vi "Simulator Thresholding.vi"(4 "RAW SICK":i16[](array[numeric]), 6 "SICK Threshold":i16, 7 "Current compass in sectors":i16) -> (0 "Actual SICK (old format)":i16[](array[numeric]), 2 "Binary SICK":i16[](array[numeric]))   [LabVIEW 2009]
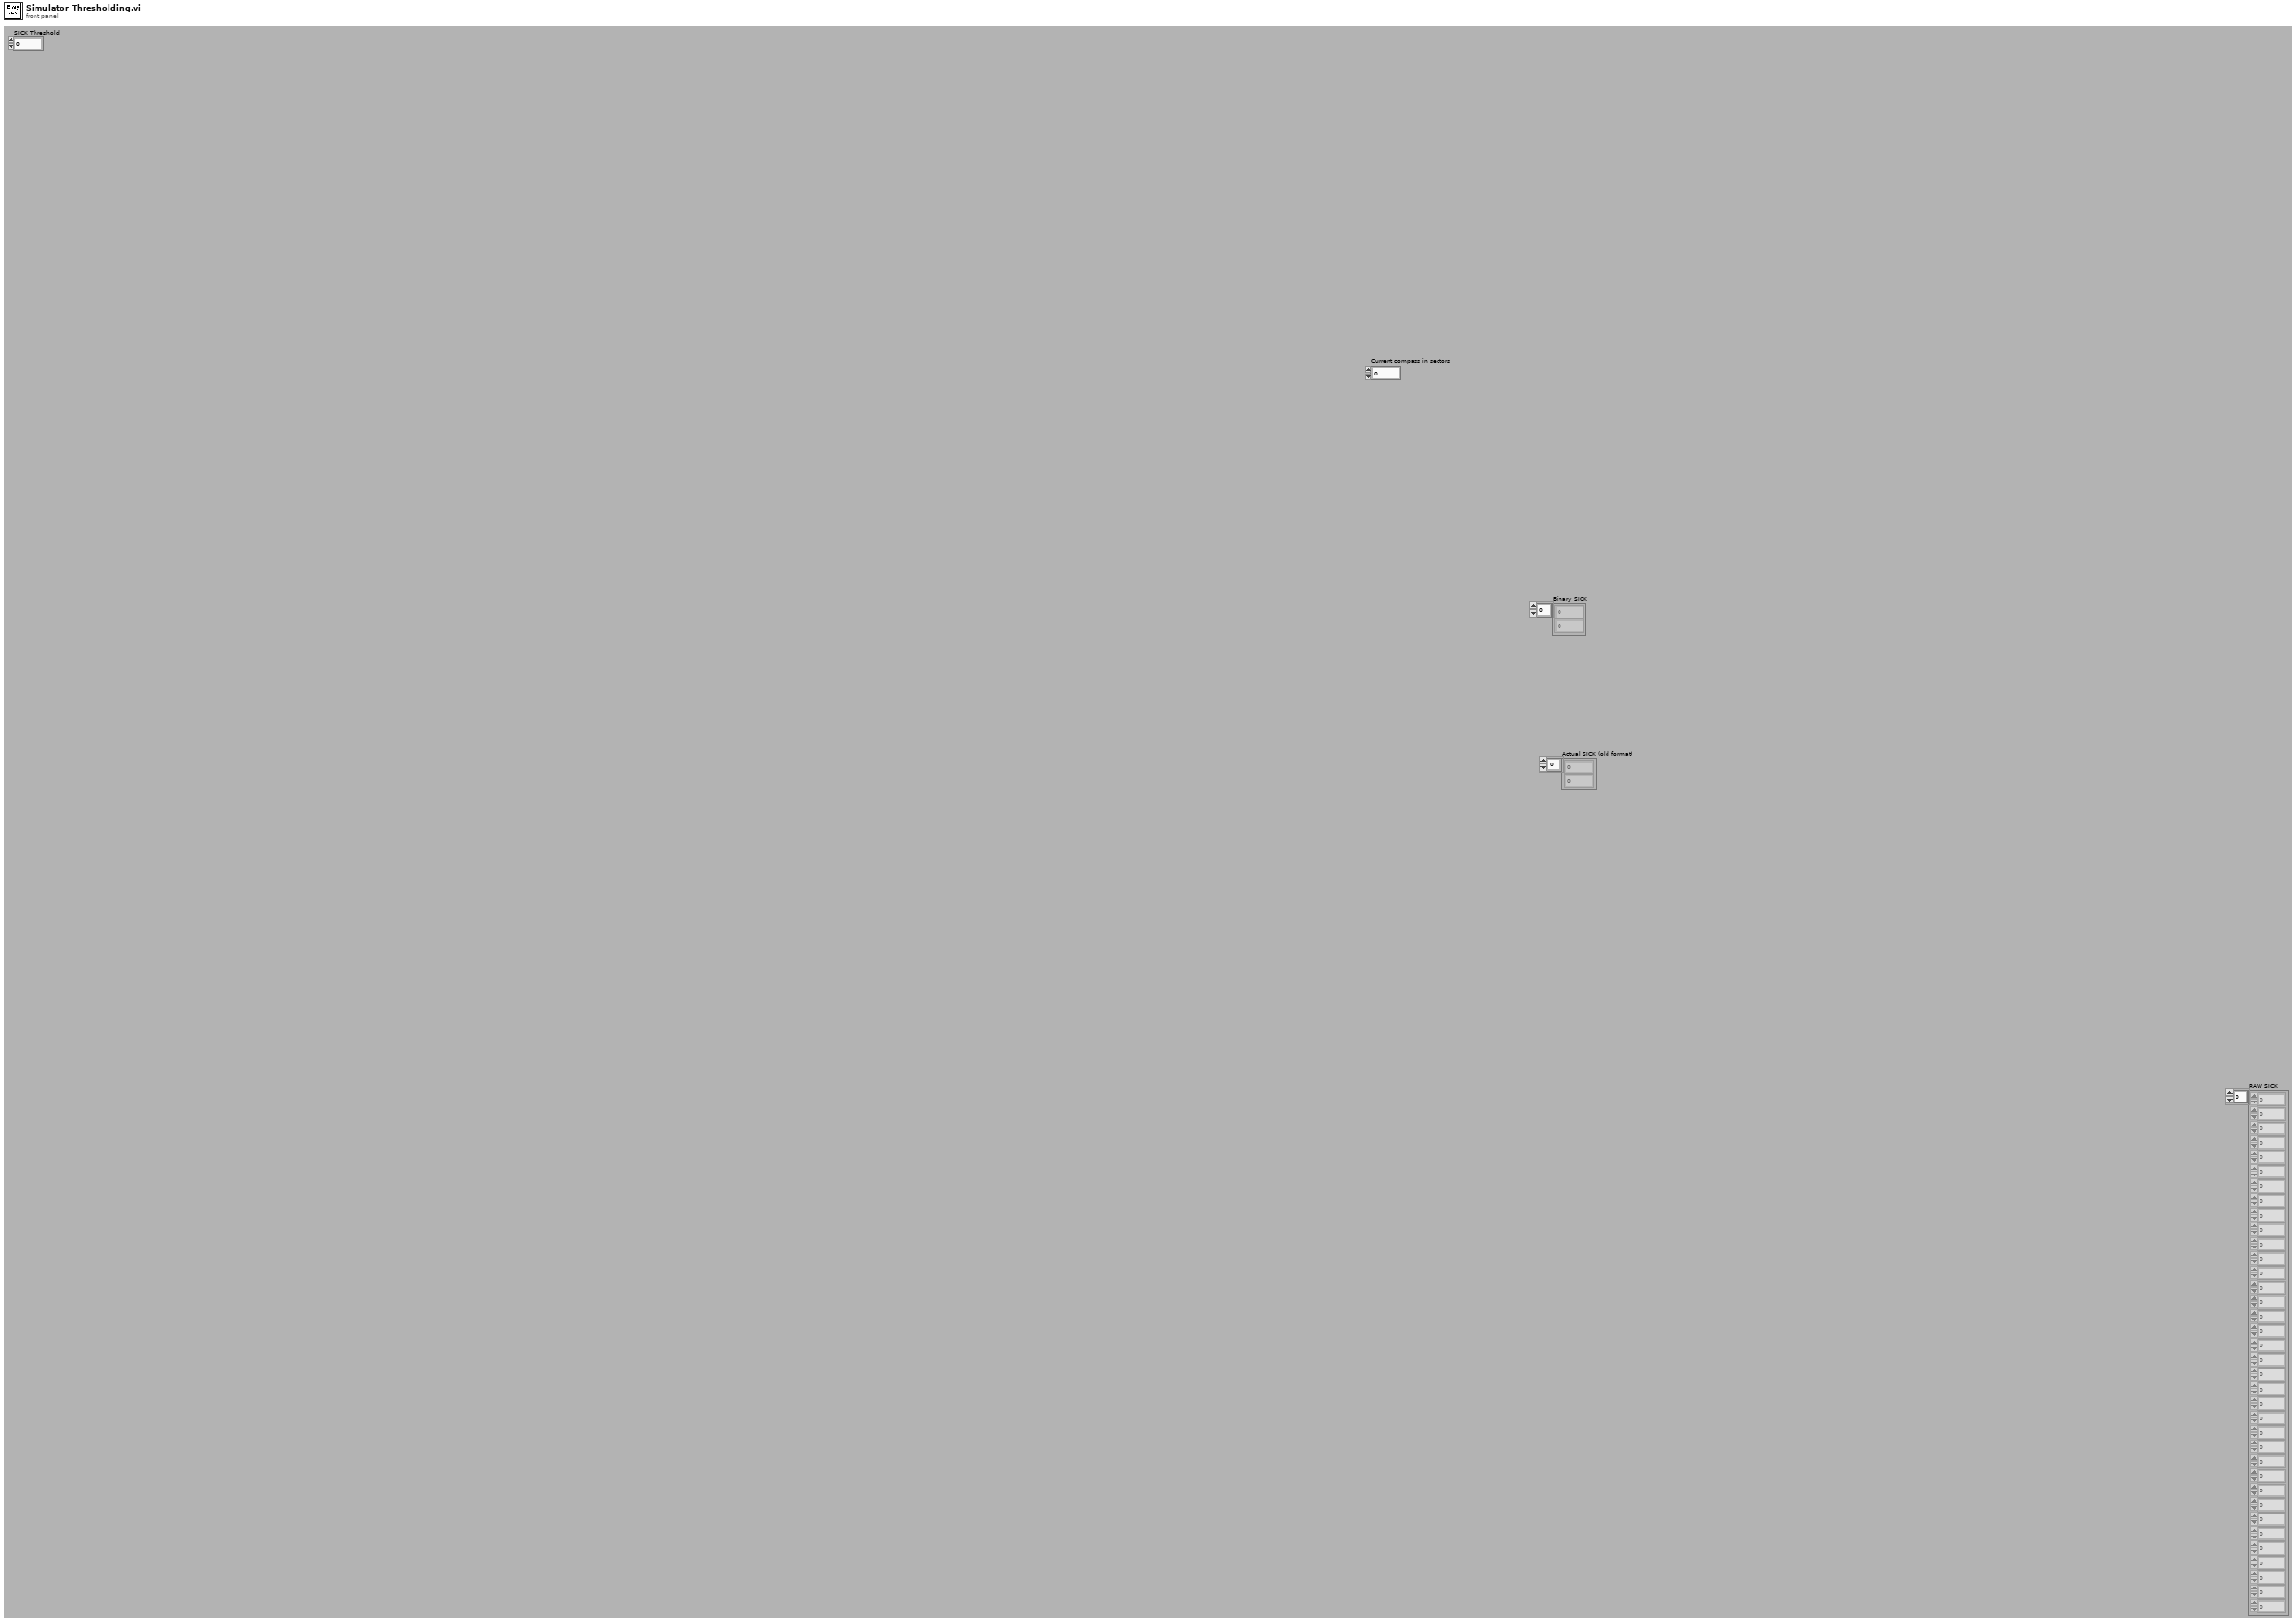
[diagram p1: front panel]
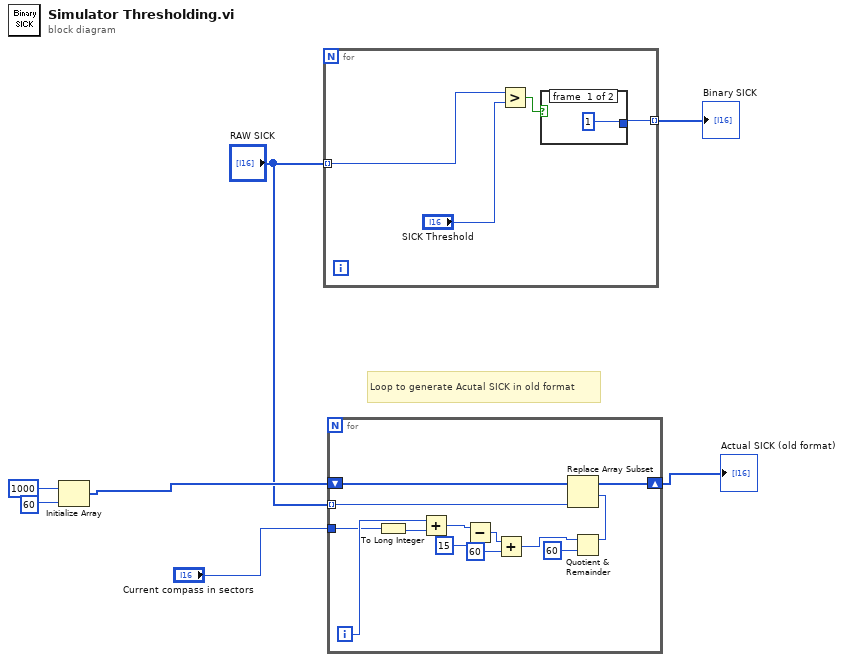
[diagram p0: block diagram]
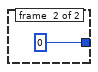
[diagram p2: hidden frame]
diagram:
  # "Loop to generate Acutal SICK in old format"
  n1 = Initialize Array(i16 1000 ("element"), 60 ("dimension size")) -> (w4:i16[])
  n2 = for {
    tunnel: "RAW SICK" -> [w11] mode=indexing
    tunnel: [w9] -> w7 mode=indexing
    n3 = Greater?(x=w11, y="SICK Threshold") -> (0:w8:bool)
    n4 = case shown="False" w8 {
      tunnel: [i16 1 i16 0] -> w9
      frame #0 {
      }
      frame #1 {
      }
    }
  }
  "Binary SICK" <- w7
  n5 = for {
    shift-right: [w25] -> w2
    shift-left: w4 -> [w26]
    tunnel: "RAW SICK" -> [w24] mode=indexing
    tunnel: "Current compass in sectors" -> [w14]
    i -> [w21]
    n6 = To Long Integer(number=w14) -> (32bit integer=w20:i32)
    n7 = Add(x=w21, y=w20) -> (x+y=w19:i32)
    n8 = Subtract(x=w19, y=15) -> (x-y=w17:i32)
    n9 = Add(x=w17, y=60) -> (x+y=w16:i32)
    n10 = Quotient & Remainder(x=w16, y=60) -> (x-y*floor(x/y)=w22:i32)  [unwired: 1 out]
    n11 = Replace Array Subset(array=w26, new element=w24, index=w22) -> (w25:i16[])
  }
  "Actual SICK (old format)" <- w2
